vi "Set Port Status.vi"(8 "error in (no error)":errorcluster, 9 "Value":string, 10 "Port":dbl, 11 "Cypress in":refnum<class "Cypress.lvclass">) -> (0 "error out":errorcluster, 3 "Cypress out":refnum<class "Cypress.lvclass">)   [LabVIEW 2020, in "Cypress.lvclass"]
doc: "Método heredado del padre con un override"
uses:
  Cypress.lvclass
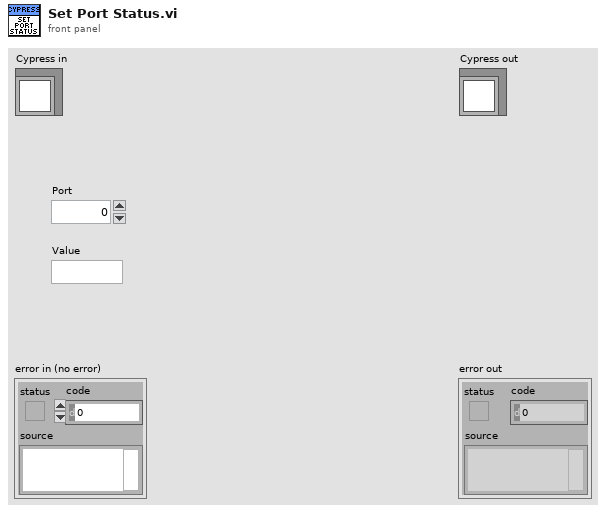
[diagram p1: front panel]
types:
  T1 = typedef "Serial device.lvclass/Brand combobox.ctl" = string
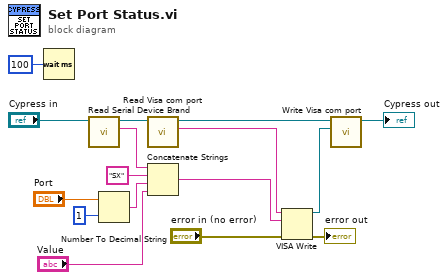
[diagram p0: block diagram]
diagram:
  n1 = Wait (ms)(milliseconds to wait=u32 100) -> ()  [unwired: 1 out]
  n2 = call-dynamic "Read Serial Device Brand.vi"("Serial device in"="Cypress in") -> ("Serial Device Brand"=w9:T1, "Serial device out"=w16:refnum<class "Cypress.lvclass">)  [unwired: 8 in, 1 out]
  n3 = Number To Decimal String(number="Port", width (-)=i16 1) -> (decimal integer string=w10:string)
  n4 = call-dynamic "Read Visa com port.vi"("Serial device in"=w16) -> ("Visa com port"=w6:string, "Serial device out"=w15:refnum<class "Cypress.lvclass">)  [unwired: 8 in, 1 out]
  n5 = Concatenate Strings(w9, "SX" ("string"), w10, "Value") -> (w5:string)
  n6 = VISA Write(VISA resource name=w6, write buffer=w5, error in (no error)="error in (no error)") -> (VISA resource name out=w4:refnum<visa-resource-name>, error out=→"error out":errorcluster)  [unwired: 1 out]
  n7 = call-dynamic "Write Visa com port.vi"("Visa com port"=w4, "Serial device in"=w15) -> ("Serial device out"=→"Cypress out":refnum<class "Cypress.lvclass">)  [unwired: 8 in, 1 out]
